vi "Register gRPC Server.vi"(8 "error in (no error)":errorcluster, 10 "gRPC ID":T1, 11 "CIFPlugin in":refnum<class "Template_Plugin.lvclass">) -> (0 "error out":errorcluster, 2 "gRPC ID Out":T1, 3 "CIFPlugin out":refnum<class "Template_Plugin.lvclass">)   [LabVIEW 2021, in "Template_Plugin.lvclass"]
uses:
  Template_Plugin.lvclass
  C:/Program Files/National Instruments/LabVIEW 2021/vi.lib/CIF Foundation/CIF Core/CIFCore/Class/CIFCorePlugin.lvclass
  <vilib>/gRPC/LabVIEW gRPC Library/Shared/grpcId.ctl
  Grpc/Template_server/RPC Service/Template/Template.lvclass
  C:/Program Files/National Instruments/LabVIEW 2021/vi.lib/gRPC/LabVIEW gRPC Servicer/ServiceBase/ServiceBase.lvclass
  <vilib>/CIF Foundation/CIF Core/CIFCore/Class/CIFCorePlugin.lvclass/CIFCorePlugin.ctl
  <vilib>/CIF Foundation/CIF Core/CIFCore/Class/Accessors/Read Register gRPC Descriptors.vi
  <vilib>/gRPC/LabVIEW gRPC Library/Server API/Server/Register Message Metadata.vi
  <vilib>/gRPC/LabVIEW gRPC Library/Server API/Server/Register Enum Metadata.vi
  Template_Plugin.lvclass/Template_Plugin.ctl
  <vilib>/CIF Foundation/CIF Core/CIFCore/Class/CIFCorePlugin.lvclass
  Grpc/Template_server/Template_server.lvlib
  <vilib>/gRPC/LabVIEW gRPC Library/grpc-lvsupport-release.lvlib
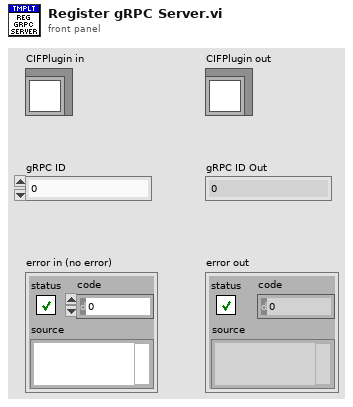
[diagram p1: front panel]
types:
  T1 = typedef "grpc-lvsupport-release.lvlib/grpcId.ctl" = u64
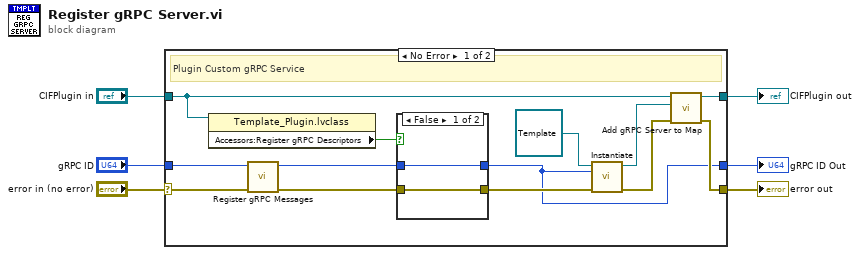
[diagram p0: block diagram]
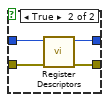
[diagram p2: hidden frame]
diagram:
  n1 = case shown="No Error" "error in (no error)" {
    selector: "error in (no error)" -> [w9 w28]
    tunnel: [w15 w28] -> w1
    tunnel: [w19 w27] -> w3
    tunnel: "CIFPlugin in" -> [w8 w27]
    tunnel: "gRPC ID" -> [w10 w26]
    tunnel: [w11 w26] -> w2
    frame No Error {
      # "Plugin Custom gRPC Service"
      n2 = property class="Template_Plugin.lvclass"(reference=w8) -> ("Accessors:Register gRPC Descriptors"=w7:bool)  [unwired: 1 in, 2 out]
      n3 = call "Register gRPC Messages.vi"("error in (no error)"=w9, "gRPC ID"=w10) -> ("error out"=w14:errorcluster, "gRPC ID Out"=w13:T1)  [unwired: 8 in]
      n4 = case shown="False" w7 {
        tunnel: w14 -> [w20 w25]
        tunnel: w13 -> [w21 w24]
        tunnel: [w20 w23] -> w12
        tunnel: [w21 w22] -> w11
        frame False {
        }
        frame True {
          n5 = call "Register Descriptors.vi"("error in (no error)"=w25, "gRPC ID"=w24) -> ("error out"=w23:errorcluster, "gRPC ID Out"=w22:T1)  [unwired: 8 in]
        }
      }
      n6 = call-dynamic "Instantiate.vi"("error in"=w12, "gRPCid"=w11, "gRPC service in"=refnum<class "Template.lvclass"> refnum ("CIF_Plugin_Core_server.lvlib:PluginCore.lvclass")) -> ("error out"=w17:errorcluster, "gRPC service out"=w16:refnum<class "Template.lvclass">)  [unwired: 7 in]
      n7 = call <vilib>:"Add gRPC Server to Map.vi"("error in (no error)"=w17, "gRPC Server Class"=w16, "CIFTemplateNode in"=w8) -> ("error out"=w15:errorcluster, "CIFTemplateNode out"=w19:refnum<class "Template_Plugin.lvclass">)  [unwired: 7 in]
    }
    frame Error {
    }
  }
  "error out" <- w1
  "CIFPlugin out" <- w3
  "gRPC ID Out" <- w2
